vi "Returning Values By Reference 2D Array Of Integers Complete.vi"() -> ()   [LabVIEW 2009, in "LabVIEWWrapper_PassingDataSampleDLL.lvlib"]
uses:
  LabVIEWWrapper_PassingDataSampleDLL.lvlib
panel:
  in  "cols":i32
  out "error out":errorcluster
  in  "error in (no error)":errorcluster
  out "Value":i32[][](array[numeric])
  in  "rows":i32
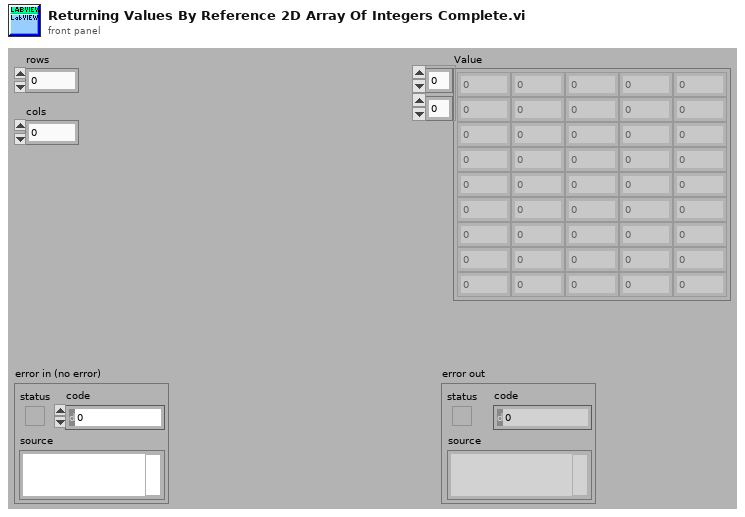
[diagram p1: front panel]
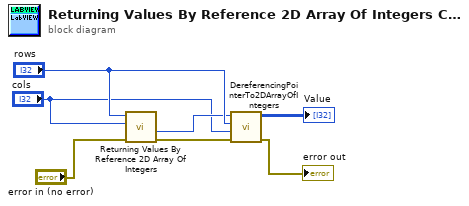
[diagram p0: block diagram]
diagram:
  n1 = call "Returning Values By Reference 2D Array Of Integers.vi"("error in (no error)"="error in (no error)", "cols"="cols", "rows"="rows") -> ("error out"=w5:errorcluster, "newArray out"=w6:i32)  [unwired: 7 in]
  n2 = call "DereferencingPointerTo2DArrayOfIntegers.vi"("error in (no error)"=w5, "Cols"="cols", "Rows"="rows", "Address (Pointer)"=w6) -> ("error out"=→"error out":errorcluster, "Value"=→"Value":i32[][])  [unwired: 6 in]
